vi "plot_normal.vi"(0 "mean":dbl, 1 "standard deviation":dbl, 2 "variance":dbl, 5 "error in (no error)":errorcluster, 10 "N":u16) -> (14 "Normal_xy":cluster{dbl[], dbl[]}, 15 "x":dbl[](array[numeric]), 16 "Normal curve":dbl[](array[numeric]), 19 "error out":errorcluster)   [LabVIEW 2020]
panel:
  in  "Tab Control":enum32{"Page 1", "Page 2"}(tab)
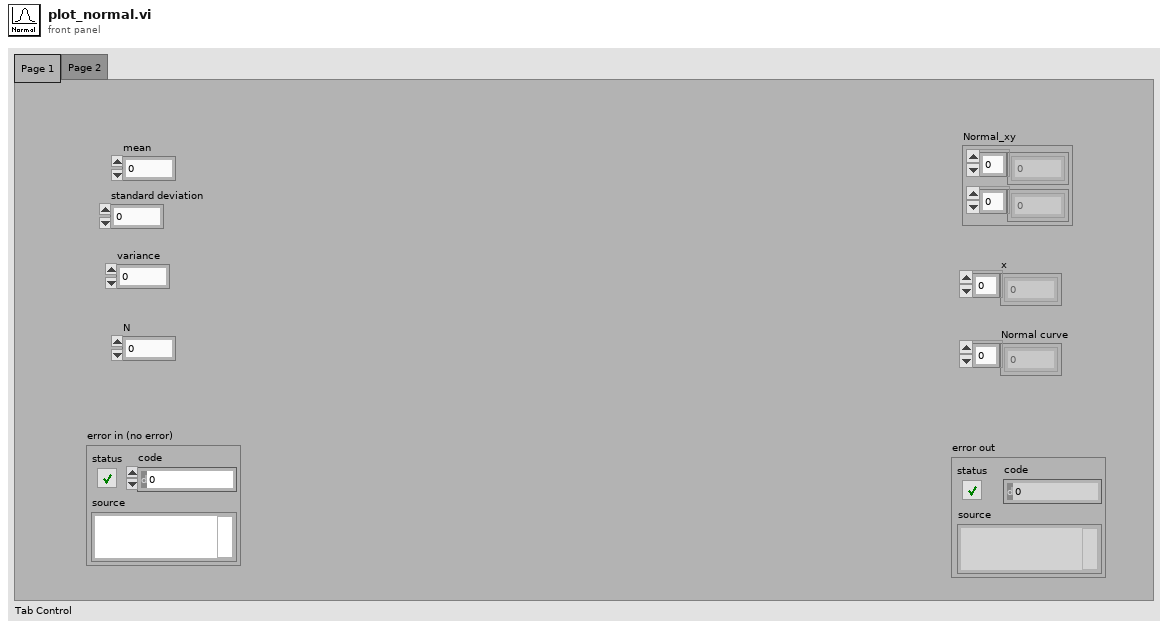
[diagram p1: front panel]
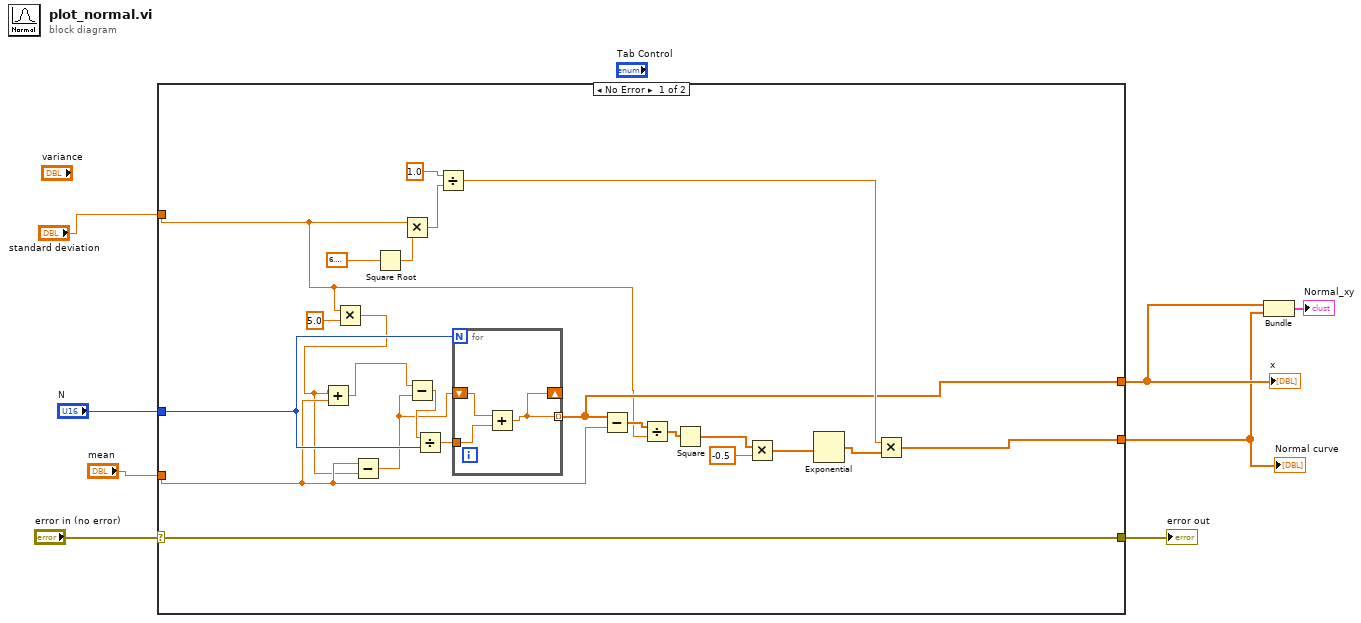
[diagram p0: block diagram]
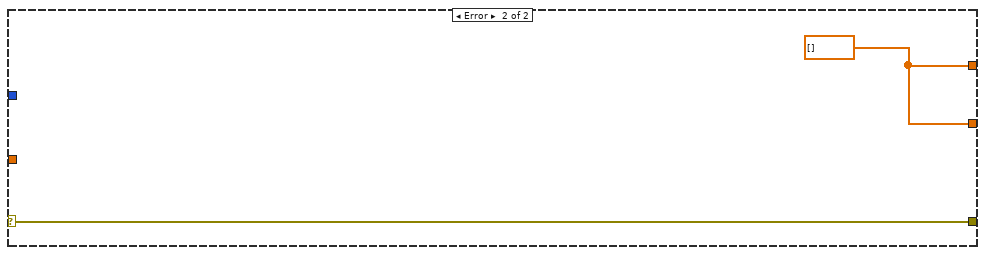
[diagram p2: hidden frame]
diagram:
  n1 = case shown="No Error" "error in (no error)" {
    selector: "error in (no error)" -> [w16 w36]
    tunnel: [w16 w36] -> w8
    tunnel: "N" -> [w31 _]
    tunnel: "standard deviation" -> [w14 _]
    tunnel: "mean" -> [w11 _]
    tunnel: [w17 w35] -> w1
    tunnel: [w15 w35] -> w3
    frame No Error {
      n2 = Multiply(x=w14, y=5.0) -> (x*y=w10:dbl)
      n3 = Add(x=w10, y=w11) -> (x+y=w12:dbl)
      n4 = Subtract(x=w11, y=w10) -> (x-y=w9:dbl)
      n5 = Square Root(x=6.283185307179586) -> (sqrt(x)=w26:dbl)
      n6 = Multiply(x=w14, y=w26) -> (x*y=w25:dbl)
      n7 = Subtract(x=w12, y=w9) -> (x-y=w30:dbl)
      n8 = Divide(x=w30, y=w31) -> (x/y=w29:dbl)
      n9 = Divide(x=1.0, y=w25) -> (x/y=w18:dbl)
      n10 = for {
        N: w31 -> [_]
        tunnel: w29 -> [w34]
        tunnel: [w32] -> w15 mode=indexing
        shift-right: [w32] -> _
        shift-left: w9 -> [w33]
        n11 = Add(x=w33, y=w34) -> (x+y=w32:dbl)
      }
      n12 = Subtract(x=w15, y=w11) -> (x-y=w24:dbl[])
      n13 = Divide(x=w24, y=w14) -> (x/y=w22:dbl[])
      n14 = Square(x=w22) -> (x^2=w21:dbl[])
      n15 = Multiply(x=w21, y=-0.5) -> (x*y=w20:dbl[])
      n16 = Exponential(1:w20) -> (0:w19:dbl[])
      n17 = Multiply(x=w18, y=w19) -> (x*y=w17:dbl[])
    }
    frame Error {
      w35 = dbl[] []
    }
  }
  "error out" <- w8
  "Normal curve" <- w1
  "x" <- w3
  n18 = Bundle(w3, w1) -> (→"Normal_xy":cluster{dbl[], dbl[]})  [unwired: 1 in]
